vi "Main PC.vi"() -> ()   [LabVIEW 2021]
panel:
  out "Array":dbl[](array[numeric])
  in  "stop":bool
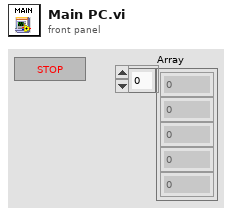
[diagram p1: front panel]
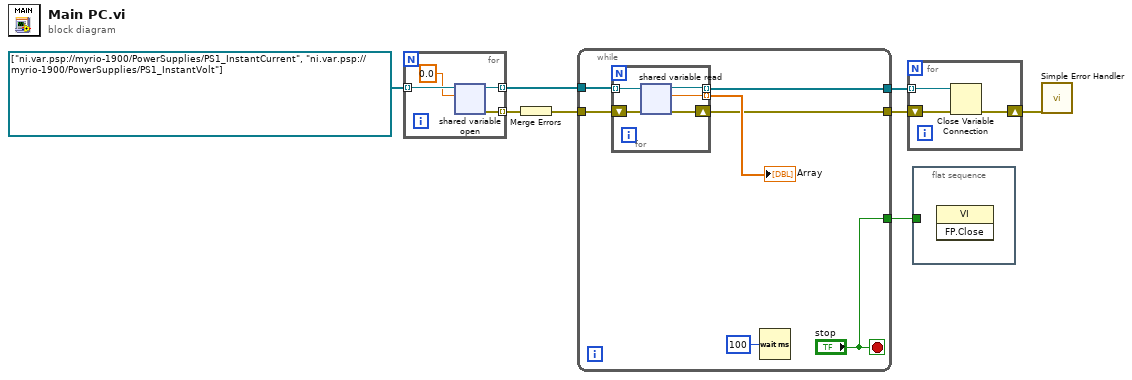
[diagram p0: block diagram]
diagram:
  n1 = for {
    tunnel: [w12] -> w7 mode=indexing
    tunnel: refnum<k21>[] ["ni.var.psp://myrio-1900/PowerSupplies/PS1_InstantCurrent", "ni.var.psp://myrio-1900/PowerSupplies/PS1_InstantVolt"] ("shared variable refnum in") -> [w11] mode=indexing
    tunnel: [w9] -> w5 mode=indexing
    n2 = shared-variable-open(w11, 0.0) -> (w12:refnum<k21>, w9:errorcluster)  [unwired: 2 in]
  }
  n3 = Merge Errors(w5) -> (w4:errorcluster)
  n4 = while {
    tunnel: ["stop"] -> w8
    tunnel: w7 -> [w17]
    tunnel: w4 -> [w16]
    tunnel: [w14] -> w3
    tunnel: [w13] -> w2
    stop <- "stop" stop-if-true
    n5 = for {
      tunnel: [w22] -> w15 mode=indexing
      shift-right: [w21] -> w13
      shift-left: w16 -> [w23]
      tunnel: w17 -> [w24] mode=indexing
      tunnel: [w20] -> w14 mode=indexing
      n6 = shared-variable-read(w24, w23) -> (w20:refnum<k21>, w21:errorcluster, w22:dbl)  [unwired: 1 out]
    }
    "Array" <- w15
    n7 = Wait (ms)(milliseconds to wait=u32 100) -> ()  [unwired: 1 out]
  }
  n8 = for {
    tunnel: w3 -> [w27] mode=indexing
    shift-right: [w25] -> w1
    shift-left: w2 -> [w26]
    n9 = Close Variable Connection(8:w26, 11:w27) -> (0:w25:errorcluster)
  }
  n10 = flat-sequence {
    tunnel: w8 -> [_]
    frame #0 {
      n11 = invoke class="VI" method="FP.Close"() -> ()  [unwired: 3 in, 3 out]
    }
  }
  n12 = call <vilib>:"Simple Error Handler.vi"("error in (no error)"=w1) -> ()  [unwired: 4 in, 5 out]
